vi "Move Camera.vi"(10 "Camera Movement":T1, 11 "Scene in":refnum<class "Scene.lvclass">) -> (3 "Scene out":refnum<class "Scene.lvclass">)   [LabVIEW 2022 SP3, in "Application.lvlib" / "Scene.lvclass"]
uses:
  Scene.lvclass
  Camera Movement.ctl
  Libraries/3D/Camera.ctl
  Scene.lvclass/Scene.ctl
  Libraries/3D/3D.lvlib
panel:
  in  "Camera Speed":sgl=2.0
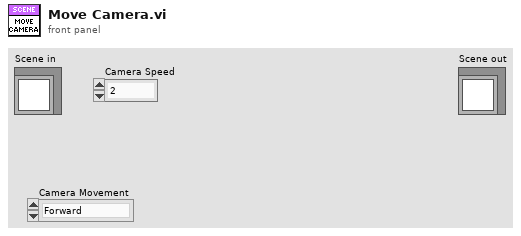
[diagram p1: front panel]
types:
  T1 = typedef "Application.lvlib/Scene.lvclass/Camera Movement.ctl" = enum16{"Forward", "Backwards", "Up", "Down", "Left", "Right", "Yaw CCW", "Yaw CW"}
  T2 = typedef "3D.lvlib/Camera.ctl" = cluster{"Field Of View":sgl, "Near Plane":sgl, "Far Plane":sgl}
  T3 = typedef "Raster.lvlib/Screen Dimensions.ctl" = cluster{"Width":u32, "Height":u32}
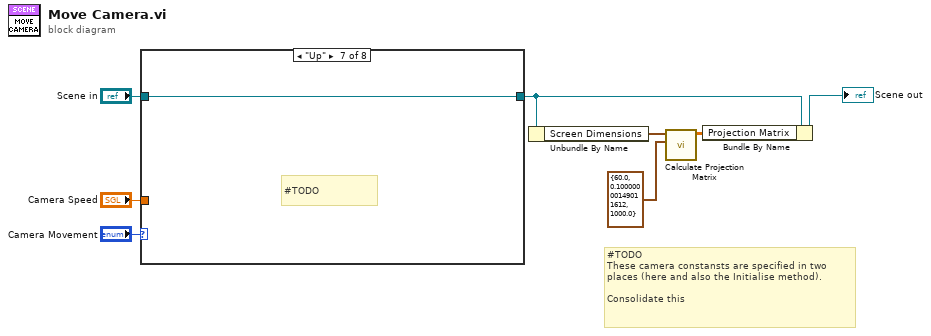
[diagram p0: block diagram]
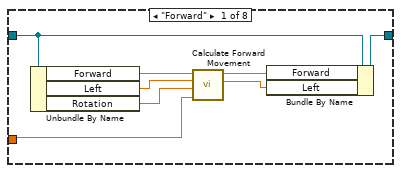
[diagram p2: hidden frame]
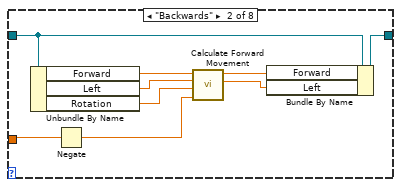
[diagram p3: hidden frame]
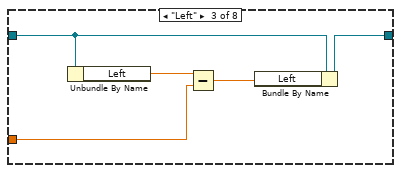
[diagram p4: hidden frame]
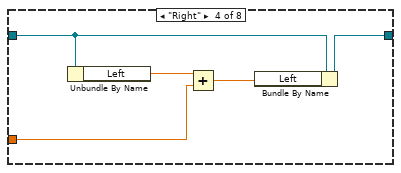
[diagram p5: hidden frame]
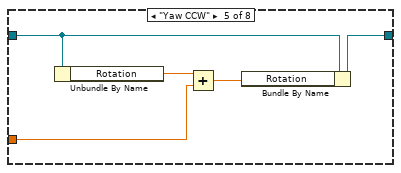
[diagram p6: hidden frame]
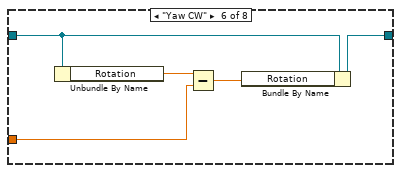
[diagram p7: hidden frame]
diagram:
  # "#TODO\nThese camera constansts are specified in two places (here and also the Initialise method).\n\nConsolidate this"
  n1 = case shown="\"Up\"" "Camera Movement" {
    tunnel: "Scene in" -> [w16 w25 w30 w35 w40 w45 w46 w47]
    tunnel: "Camera Speed" -> [w11 w20 w29 w34 w39 w44 _ _]
    tunnel: [w13 w22 w26 w31 w36 w41 w46 w47] -> w6
    frame "Forward" {
      n2 = Unbundle By Name(w16) -> ("Forward"=w15:sgl, "Left"=w10:sgl, "Rotation"=w9:sgl)
      n3 = call "Calculate Forward Movement.vi"("Camera Speed"=w11, "Rotation"=w9, "Previous Left"=w10, "Previous Forward"=w15) -> ("Next Left"=w12:sgl, "Next Forward"=w14:sgl)  [unwired: 6 in]
      n4 = Bundle By Name(cluster=w16, "Forward"=w14, "Left"=w12) -> (w13:refnum<class "Scene.lvclass">)
    }
    frame "Backwards" {
      n5 = Unbundle By Name(w25) -> ("Forward"=w24:sgl, "Left"=w19:sgl, "Rotation"=w18:sgl)
      n6 = Negate(x=w20) -> (-x=w17:sgl)
      n7 = call "Calculate Forward Movement.vi"("Camera Speed"=w17, "Rotation"=w18, "Previous Left"=w19, "Previous Forward"=w24) -> ("Next Left"=w21:sgl, "Next Forward"=w23:sgl)  [unwired: 6 in]
      n8 = Bundle By Name(cluster=w25, "Forward"=w23, "Left"=w21) -> (w22:refnum<class "Scene.lvclass">)
    }
    frame "Left" {
      n9 = Unbundle By Name(w30) -> ("Left"=w28:sgl)
      n10 = Subtract(x=w28, y=w29) -> (x-y=w27:sgl)
      n11 = Bundle By Name(cluster=w30, "Left"=w27) -> (w26:refnum<class "Scene.lvclass">)
    }
    frame "Right" {
      n12 = Unbundle By Name(w35) -> ("Left"=w33:sgl)
      n13 = Add(x=w33, y=w34) -> (x+y=w32:sgl)
      n14 = Bundle By Name(cluster=w35, "Left"=w32) -> (w31:refnum<class "Scene.lvclass">)
    }
    frame "Yaw CCW" {
      n15 = Unbundle By Name(w40) -> ("Rotation"=w38:sgl)
      n16 = Add(x=w38, y=w39) -> (x+y=w37:sgl)
      n17 = Bundle By Name(cluster=w40, "Rotation"=w37) -> (w36:refnum<class "Scene.lvclass">)
    }
    frame "Yaw CW" {
      n18 = Unbundle By Name(w45) -> ("Rotation"=w43:sgl)
      n19 = Subtract(x=w43, y=w44) -> (x-y=w42:sgl)
      n20 = Bundle By Name(cluster=w45, "Rotation"=w42) -> (w41:refnum<class "Scene.lvclass">)
    }
    frame "Up" {
      # "#TODO"
    }
    frame "Down" {
      # "#TODO"
    }
  }
  n21 = Unbundle By Name(w6) -> ("Screen Dimensions"=w8:T3)
  n22 = call "Calculate Projection Matrix.vi"("Camera"=T2 {"Field Of View"=60.0, "Near Plane"=0.1, "Far Plane"=1000.0}, "Screen Dimensions"=w8) -> ("Projection Matrix"=w7:sgl[][])  [unwired: 9 in]
  n23 = Bundle By Name(cluster=w6, "Projection Matrix"=w7) -> (→"Scene out":refnum<class "Scene.lvclass">)
